vi "Random Number Within Range__ogtk.vi"   [LabVIEW 2018]
doc: "Generates a <b>Random Number</b> between <b>High</b> and <b>Low</b> inputs. Prechecks data to ensure that <b>High</b> is greater than <b>Low</b>."
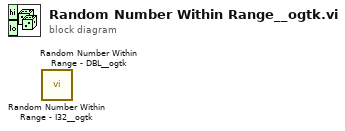
[diagram p0: block diagram]
diagram:
  n1 = call <userlib>:"Random Number Within Range - I32__ogtk.vi"() -> ()  [unwired: 5 in, 1 out]
  n2 = call <userlib>:"Random Number Within Range - DBL__ogtk.vi"() -> ()  [unwired: 5 in, 1 out]
